vi "Revert to Scan Mode.vi"(8 "error in":errorcluster, 10 "Target IP Address":string, 11 "Slave Ref":variant) -> (0 "error out":errorcluster)   [LabVIEW 2019, in "SEECD System Explorer.lvlib"]
uses:
  SEECD System Explorer.lvlib
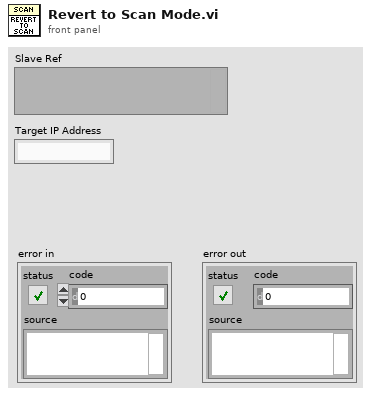
[diagram p1: front panel]
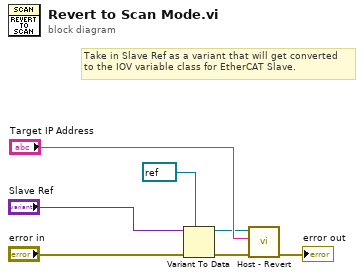
[diagram p0: block diagram]
diagram:
  # "Take in Slave Ref as a variant that will get converted\nto the IOV variable class for EtherCAT Slave."
  n1 = Variant To Data(error in="error in", type=refnum<k21> refnum ("Slave Ref 2"), Variant="Slave Ref") -> (data=w1:refnum<k21>, error out=w4:errorcluster)
  n2 = call "Host - Revert.vi"("error in"=w4, "Target IP Address in"="Target IP Address", "Slave Ref in"=w1) -> ("error out"=→"error out":errorcluster)  [unwired: 6 in, 2 out]
